vi "Práctica_04.vi"() -> ()   [LabVIEW 2020]
uses:
  <vilib>/express/express shared/transition.llb/Dynamic To Waveform Array.vi
  <vilib>/express/express signal manip/GetorSetDDTAttributes/Set DDT Attributes/SetT0.vi
  <vilib>/express/express shared/transition.llb/Waveform Array To Dynamic.vi
  <vilib>/express/express signal manip/GetorSetDDTAttributes/Set DDT Attributes/Set DDT Properties.xnode
panel:
  in  "Activar escritura de datos":bool=TRUE caption="Flush? (T)"
  out "Valor Mínimo":dbl
  out "Valor Máximo":dbl
  in  "stop":bool
  out "Waveform Chart":dynamicdata(graph)
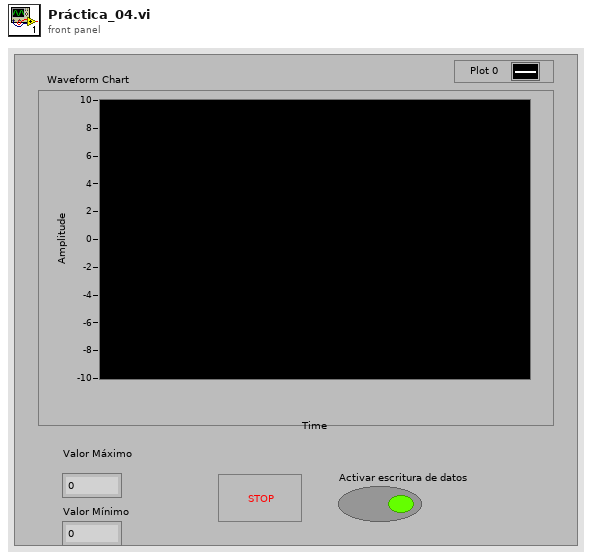
[diagram p1: front panel]
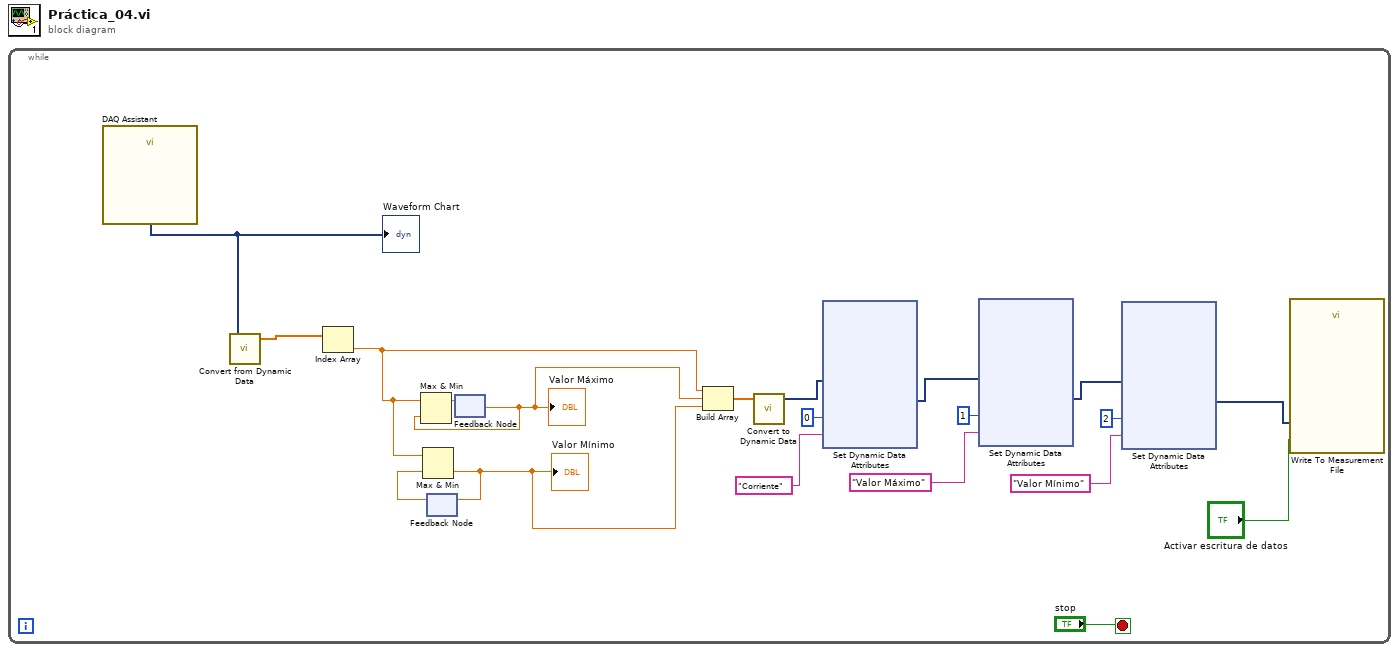
[diagram p0: block diagram]
diagram:
  n1 = while {
    stop <- "stop" stop-if-true
    n2 = call "DAQ Assistant"() -> ("data"=w20:dynamicdata)  [unwired: 17 in, 2 out]
    "Waveform Chart" <- w20
    n3 = call "Convert from Dynamic Data"("Dynamic Data Type"=w20) -> ("Array"=w19:dbl[])  [unwired: 3 in]
    n4 = Index Array "Index Array"(array=w19) -> (element=w3:dbl)  [unwired: 1 in]
    n5 = feedback #1() -> (w16:dbl)  [unwired: 1 in]
    n6 = Max & Min(x=w3, y=w16) -> (min(x,y)=w1:dbl)  [unwired: 1 out]
    "Valor Mínimo" <- w1
    n7 = feedback-in #1(w1) -> ()
    n8 = feedback #2() -> (w2:dbl)  [unwired: 1 in]
    "Valor Máximo" <- w2
    n9 = Max & Min(x=w3, y=w2) -> (max(x,y)=w17:dbl)  [unwired: 1 out]
    n10 = feedback-in #2(w17) -> ()
    n11 = Build Array(w3, w2, w1) -> (w9:dbl[])
    n12 = call "Convert to Dynamic Data"("Array"=w9) -> ("Dynamic Data Type"=w8:dynamicdata)  [unwired: 3 in]
    n13 = xnode "Set Dynamic Data Attributes"("Signals In"=w8, "Signal Index"=0, "Signal Name"="Corriente") -> ("Signals Out"=w14:dynamicdata)  [unwired: 1 in, 1 out]
    n14 = xnode "Set Dynamic Data Attributes"("Signals In"=w14, "Signal Index"=1, "Signal Name"="Valor Máximo") -> ("Signals Out"=w12:dynamicdata)  [unwired: 1 in, 1 out]
    n15 = xnode "Set Dynamic Data Attributes"("Signals In"=w12, "Signal Index"=2, "Signal Name"="Valor Mínimo") -> ("Signals Out"=w10:dynamicdata)  [unwired: 1 in, 1 out]
    n16 = call "Write To Measurement File"("Signals"=w10, "Flush? (T)"="Activar escritura de datos") -> ()  [unwired: 15 in, 3 out]
  }
